vi "Split (multiple).vi"(8 "error in (no error)":errorcluster, 9 "fractional index":dbl, 11 "XY-data":cluster{"X-array":dbl[], "Y-array":dbl[]}[](array[cluster]) {"Y-array" format="%.2p"; "X-array" format="%.2p"}) -> (0 "error out":errorcluster, 2 "XY-data (B) out":cluster{"X-array":dbl[], "Y-array":dbl[]}[](array[cluster]), 3 "XY-data (A) out":cluster{"X-array":dbl[], "Y-array":dbl[]}[](array[cluster]))   [LabVIEW 2019, in "xy_utilities.lvlib"]
doc: "Divides <B>XY-Data</B> at <b>index</b> (in units of the x array) and returns <B>XY-Data A</B> and <B>XY-Data B</B>.\n\nThe element at <b>index</b> will be at the beginning of <B>XY-Data B</B>\n\nWire data to the data input to determine the polymorphic instance to use or manually select the instance."
uses:
  xy_utilities.lvlib
  Sort.vi
  Sort (single).vi
  <userlib>/_OpenG.lib/array/array.llb/Sort Array__ogtk.vi
  <userlib>/_OpenG.lib/array/array.llb/Sort 1D Array (DBL)__ogtk.vi
  <userlib>/_OpenG.lib/array/array.llb/Reorder Array2__ogtk.vi
  <userlib>/_OpenG.lib/array/array.llb/Reorder 1D Array2 (DBL)__ogtk.vi
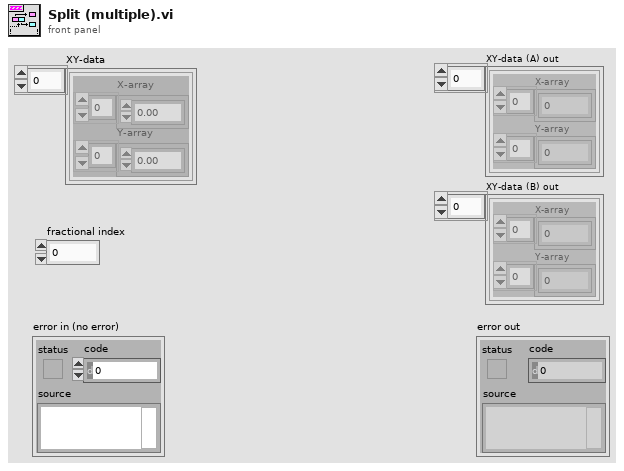
[diagram p1: front panel]
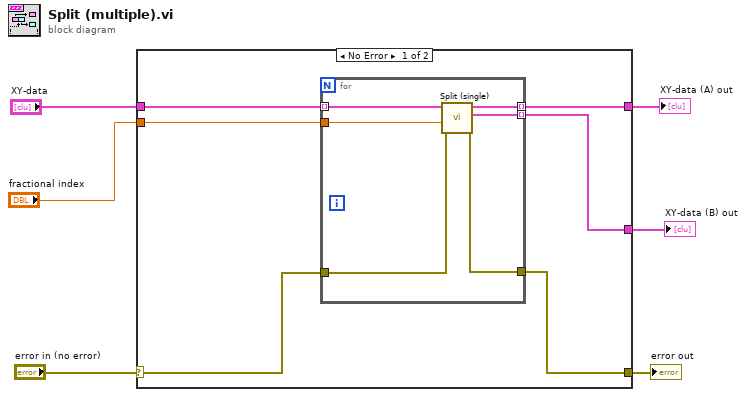
[diagram p0: block diagram]
diagram:
  n1 = case shown="No Error" "error in (no error)" {
    selector: "error in (no error)" -> [w10 w20]
    tunnel: [w9 w20] -> w5
    tunnel: "XY-data" -> [w12 w19]
    tunnel: [w11 w19] -> w4
    tunnel: [w8 _] -> w2
    tunnel: "fractional index" -> [w7 _]
    frame No Error {
      n2 = for {
        tunnel: w12 -> [w15] mode=indexing
        tunnel: [w18] -> w11 mode=indexing
        tunnel: w10 -> [w17]
        tunnel: [w16] -> w9
        tunnel: [w14] -> w8 mode=indexing
        tunnel: w7 -> [w13]
        n3 = call "Split (single).vi"("error in (no error)"=w17, "fractional index"=w13, "XY-data"=w15) -> ("error out"=w16:errorcluster, "XY-data (B) out"=w14:cluster{"X-array":dbl[], "Y-array":dbl[]}, "XY-data (A) out"=w18:cluster{"X-array":dbl[], "Y-array":dbl[]})  [unwired: 6 in]
      }
    }
    frame Error {
    }
  }
  "error out" <- w5
  "XY-data (A) out" <- w4
  "XY-data (B) out" <- w2
